vi "SDSU_GetClkList.vi"(9 "mux name":string, 10 "Table":string[][](table)) -> (1 "clks str":string, 2 "cloks":string[][](array[string]), 5 "mux num":string, 7 "board num":string)   [LabVIEW 2016]
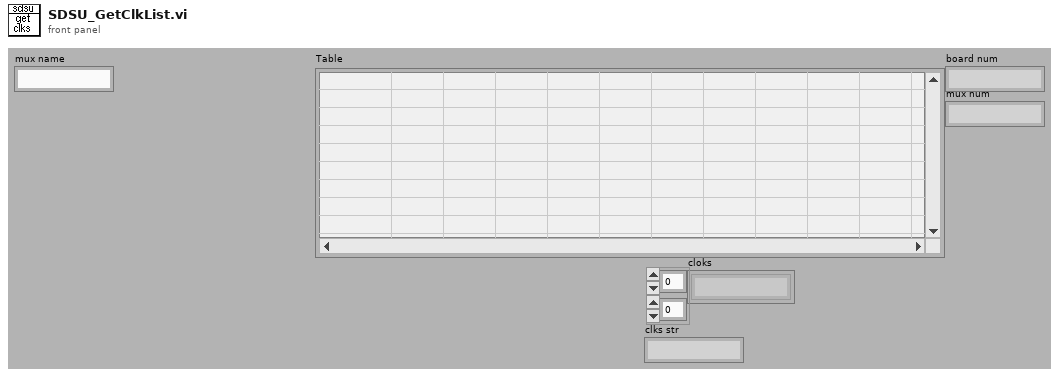
[diagram p1: front panel]
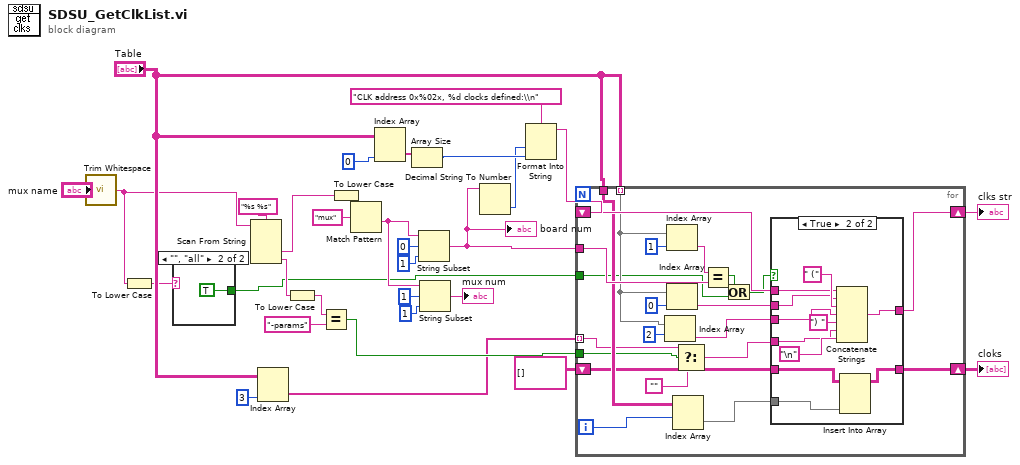
[diagram p0: block diagram]
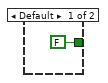
[diagram p2: hidden frame]
diagram:
  n1 = call <vilib>:"Trim Whitespace.vi"("string"="mux name") -> ("trimmed string"=w3:string)  [unwired: 1 in]
  n2 = To Lower Case(string=w3) -> (all lower case string=w1:string)
  n3 = case shown="\"\", \"all\"" w1 {
    tunnel: [FALSE TRUE] -> w2
    frame Default {
    }
    frame "", "all" {
    }
  }
  n4 = Scan From String(format string="%s %s", input string=w3) -> (output 1=w12:string, output 2=w11:string)  [unwired: 2 in, 5 out]
  n5 = Index Array(array="Table", index (col)=3 ("disabled index (col)")) -> (element=w5:string[])  [unwired: 1 in]
  n6 = To Lower Case(string=w11) -> (all lower case string=w10:string)
  n7 = Equal?(x=w10, y="-params") -> (x = y?=w6:bool)
  n8 = To Lower Case(string=w12) -> (all lower case string=w21:string)
  n9 = Match Pattern(string=w21, regular expression="mux") -> (after substring=w25:string)  [unwired: 4 out]
  n10 = Index Array(array="Table", index (col)=0 ("index")) -> (element=w18:string[])  [unwired: 1 in]
  n11 = Array Size(array=w18) -> (size(s)=w17:i32)
  n12 = String Subset(string=w25, offset (0)=0, length (rest)=1 ("length (rest)")) -> (substring=w15:string)
  "board num" <- w15
  n13 = String Subset(string=w25, offset (0)=1, length (rest)=1 ("length (rest)")) -> (substring=→"mux num":string)
  n14 = Decimal String To Number(string=w15) -> (number=w14:i32)  [unwired: 3 out]
  n15 = Format Into String(format string="CLK address 0x%02x, %d clocks defined:\\n", w14, w17) -> (resulting string=w16:string)  [unwired: 2 in, 1 out]
  n16 = for {
    shift-right: [w49] -> w27
    shift-left: w16 -> [w48]
    tunnel: w15 -> [w54]
    tunnel: "Table" -> [w47] mode=indexing
    tunnel: "Table" -> [w45]
    shift-right: [w42] -> w28
    shift-left: string[][] [] -> [w41]
    tunnel: w6 -> [w39]
    tunnel: w5 -> [w38] mode=indexing
    tunnel: w2 -> [w35]
    i -> [w44]
    n17 = Index Array(array=w47, index=2) -> (element=w50:string)
    n18 = Index Array(array=w47, index=1) -> (element=w46:string)
    n19 = Index Array(array=w47, index=0) -> (element=w51:string)
    n20 = Index Array(array=w45, index (row)=w44) -> (element=w43:string[])  [unwired: 1 in]
    n21 = Select(t=w38, s=w39, f="") -> (s? t:f=w37:string)
    n22 = Equal?(x=w46, y=w54) -> (x = y?=w36:bool)
    n23 = Or(x=w36, y=w35) -> (x .or. y?=w34:bool)
    n24 = case shown="True" w34 {
      tunnel: w51 -> [_ w64]
      tunnel: w50 -> [_ w63]
      tunnel: [w57 w66] -> w49
      tunnel: w48 -> [w57 w65]
      tunnel: w43 -> [_ w62]
      tunnel: [w56 w61] -> w42
      tunnel: w41 -> [w56 w60]
      tunnel: w37 -> [_ w58]
      frame False {
      }
      frame True {
        n25 = Concatenate Strings(w65, w64, " (" ("string"), w63, ") " ("string"), w58, "\n") -> (w66:string)
        n26 = Insert Into Array(array=w60, new element=w62) -> (w61:string[][])  [unwired: 2 in]
      }
    }
  }
  "cloks" <- w28
  "clks str" <- w27
